vi "As PropertyObject.vi"(8 "error in (no error)":errorcluster, 11 "Step in":refnum<class "Step.lvclass">) -> (0 "error out":errorcluster, 2 "PropertyObject":refnum<k7>, 3 "Step out":refnum<class "Step.lvclass">)   [LabVIEW 2020, in "TSnax.lvlib" / "Step.lvclass"]
uses:
  Step.lvclass
  Step.lvclass/Step.ctl
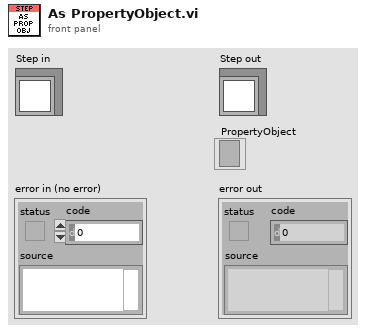
[diagram p1: front panel]
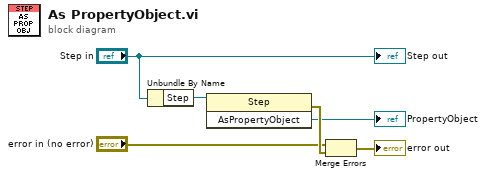
[diagram p0: block diagram]
diagram:
  n1 = Unbundle By Name("Step in") -> ("Step"=w3:refnum<k7>)
  n2 = invoke class="Step" method="AsPropertyObject"(reference=w3) -> (error out=w6:errorcluster, "AsPropertyObject"=→"PropertyObject":refnum<k7>)  [unwired: 2 in, 1 out]
  n3 = Merge Errors("error in (no error)", w6) -> (→"error out":errorcluster)
  "Step out" <- "Step in"
